vi "Cleanup.vi"(8 "error in (no error)":errorcluster, 11 "High Res Arithmetic in":refnum<class "High Res Arithmetic.lvclass">) -> (0 "error out":errorcluster, 3 "High Res Arithmetic out":refnum<class "High Res Arithmetic.lvclass">)   [LabVIEW 2021, in "High Res Arithmetic.lvclass"]
uses:
  High Res Arithmetic.lvclass
  High Res Arithmetic.lvclass/High Res Arithmetic.ctl
  <vilib>/gmath/NI_Gmath.lvlib
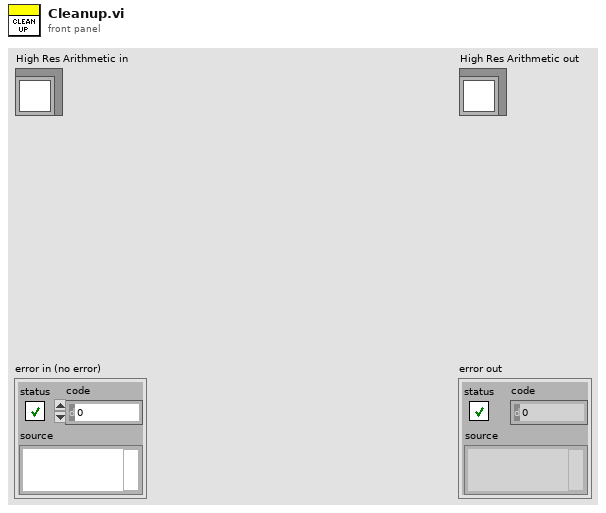
[diagram p1: front panel]
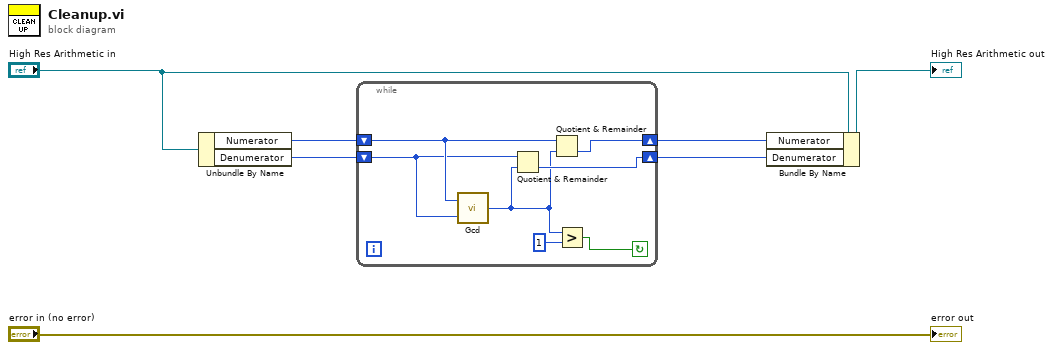
[diagram p0: block diagram]
diagram:
  n1 = Unbundle By Name("High Res Arithmetic in") -> ("Numerator"=w4:i64, "Denumerator"=w3:i64)
  n2 = while {
    shift-right: [w13] -> w2
    shift-left: w4 -> [w14]
    shift-right: [w11] -> w1
    shift-left: w3 -> [w12]
    stop <- w8 continue-if-true
    n3 = call <vilib>:"Gcd.vi"("y"=w12, "x"=w14) -> ("gcd(x,y)"=w10:i32)
    n4 = Quotient & Remainder(x=w12, y=w10) -> (floor(x/y)=w11:i64)  [unwired: 1 out]
    n5 = Quotient & Remainder(x=w14, y=w10) -> (floor(x/y)=w13:i64)  [unwired: 1 out]
    n6 = Greater?(x=w10, y=1) -> (0:w8:bool)
  }
  n7 = Bundle By Name(cluster="High Res Arithmetic in", "Numerator"=w2, "Denumerator"=w1) -> (→"High Res Arithmetic out":refnum<class "High Res Arithmetic.lvclass">)
  "error out" <- "error in (no error)"
